vi "generator_of_pickup_code.vi"(8 "row":i32, 9 "column":i32, 10 "recipient_email":string, 11 "location_of_locker_for_recipient":u16) -> (3 "pick-up code":string)   [LabVIEW 2023]
uses:
  <vilib>/numeric/Random Number (Range) U64.vi
  <vilib>/numeric/sub_Random U32.vi
  <vilib>/Utility/file.llb/Read Delimited Spreadsheet (string).vi
  <vilib>/Utility/file.llb/Write Delimited Spreadsheet (string).vi
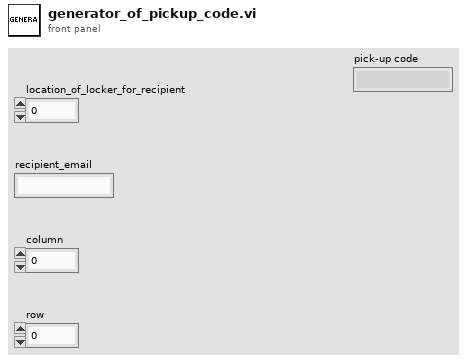
[diagram p1: front panel]
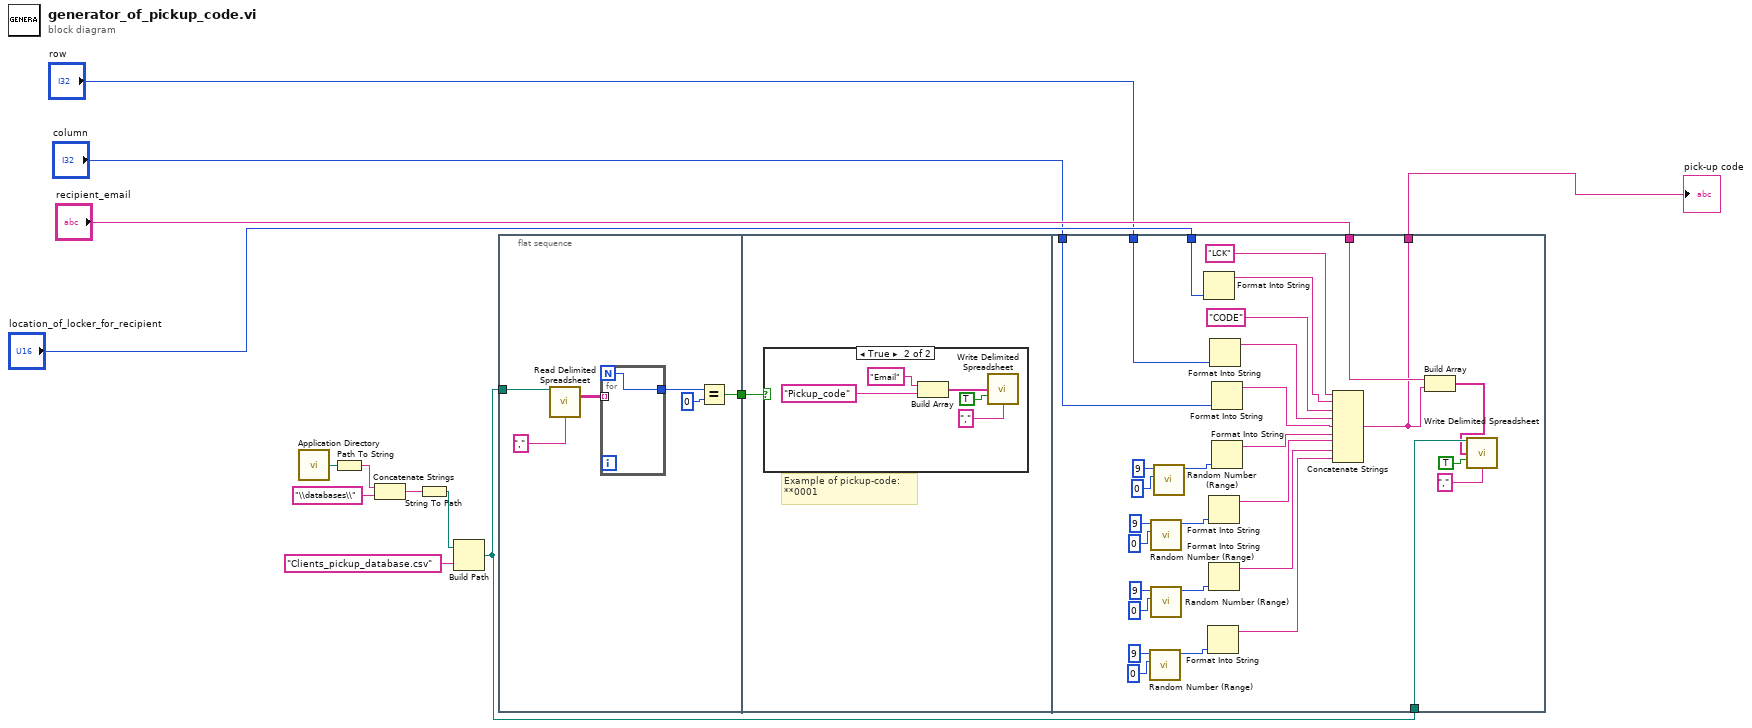
[diagram p0: block diagram]
diagram:
  n1 = call <vilib>:"Application Directory.vi"() -> ("Application Directory"=w8:path)
  n2 = Path To String(path=w8) -> (string=w7:string)
  n3 = Concatenate Strings(w7, "\\databases\\") -> (w5:string)
  n4 = String To Path(string=w5) -> (path=w4:path)
  n5 = Build Path(base path=w4, name or relative path="Clients_pickup_database.csv") -> (appended path=w10:path)
  n6 = flat-sequence {
    tunnel: w10 -> [w17]
    tunnel: [w15] -> w13
    tunnel: w13 -> [w21]
    tunnel: w10 -> [w35]
    tunnel: "recipient_email" -> [w31]
    tunnel: "location_of_locker_for_recipient" -> [w30]
    tunnel: "row" -> [w29]
    tunnel: "column" -> [w28]
    tunnel: [w27] -> w1
    frame #0 {
      n7 = call-poly <vilib>:"Read Delimited Spreadsheet.vi"("file path (dialog if empty)"=w17, "delimiter (\\t)"="," ("delimiter (\\t)")) -> ("all rows"=w18:string[][])  [unwired: 8 in, 5 out]
      n8 = for {
        N -> [w20]
        tunnel: w18 -> [_] mode=indexing
        tunnel: [w20] -> w14
      }
      n9 = Equal?(x=w14, y=0) -> (x = y?=w15:bool)
    }
    frame #1 {
      # "Example of pickup-code:\n**0001"
      n10 = case shown="True" w21 {
        frame False {
        }
        frame True {
          n11 = Build Array("Email", "Pickup_code") -> (w23:string[])
          n12 = call-poly <vilib>:"Write Delimited Spreadsheet.vi"("1D data"=w23, "append to file? (new file:F)"=TRUE, "delimiter (\\t)"="," ("delimiter (\\t)")) -> ()  [unwired: 11 in, 2 out]
        }
      }
    }
    frame #2 {
      n13 = call-poly <vilib>:"Random Number (Range).vi"("lower bound (0)"=u64 0, "upper bound (100)"=u64 9) -> ("number"=w49:u64)  [unwired: 9 in]
      n14 = call-poly <vilib>:"Random Number (Range).vi"("lower bound (0)"=u64 0, "upper bound (100)"=u64 9) -> ("number"=w47:u64)  [unwired: 9 in]
      n15 = call-poly <vilib>:"Random Number (Range).vi"("lower bound (0)"=u64 0, "upper bound (100)"=u64 9) -> ("number"=w48:u64)  [unwired: 9 in]
      n16 = call-poly <vilib>:"Random Number (Range).vi"("lower bound (0)"=u64 0, "upper bound (100)"=u64 9) -> ("number"=w46:u64)  [unwired: 9 in]
      n17 = Format Into String(w30) -> (resulting string=w50:string)  [unwired: 3 in, 1 out]
      n18 = Format Into String(w49) -> (resulting string=w56:string)  [unwired: 3 in, 1 out]
      n19 = Format Into String(w47) -> (resulting string=w54:string)  [unwired: 3 in, 1 out]
      n20 = Format Into String(w48) -> (resulting string=w55:string)  [unwired: 3 in, 1 out]
      n21 = Format Into String(w29) -> (resulting string=w51:string)  [unwired: 3 in, 1 out]
      n22 = Format Into String(w28) -> (resulting string=w52:string)  [unwired: 3 in, 1 out]
      n23 = Format Into String(w46) -> (resulting string=w53:string)  [unwired: 3 in, 1 out]
      n24 = Concatenate Strings "Concatenate Strings"("LCK", w50, "CODE", w51, w52, w53, w54, w55, w56) -> (w27:string)
      n25 = Build Array(w31, w27) -> (w32:string[])
      n26 = call-poly <vilib>:"Write Delimited Spreadsheet.vi"("file path (dialog if empty)"=w35, "1D data"=w32, "append to file? (new file:F)"=TRUE, "delimiter (\\t)"="," ("delimiter (\\t)")) -> ()  [unwired: 10 in, 2 out]
    }
  }
  "pick-up code" <- w1
